vi "rtc.vi"(8 "per":dbl, 9 "Altitude (Z)":dbl(slide)=2.0 scale=0.0..10.0, 10 "Longitude (Y)":dbl(slide) scale=0.0..10.0, 11 "Latitude (X)":dbl(slide)) -> (0 "yaw":dbl, 1 "Zo":dbl, 2 "Yo":dbl, 3 "Xo":dbl, 4 "pitch":dbl, 6 "h":dbl)   [LabVIEW 2015]
uses:
  <vilib>/imath/engines/lvmath2/RunTimeEngine/Managers/WorkSpace/UID Generator.vi
  <vilib>/imath/engines/lvmath2/RunTimeEngine/BuiltInFunctions/pause/NIMS_pause(S).vi
  <vilib>/imath/engines/lvmath2/RunTimeEngine/RunTimeType/NIMS_RunTimeType_From StrictType (excl LVString).vi
  <instcachedir>/0/NIMS_RunTimeType_From StrictType (excl LVString)_EB1C38A9BC5048DA9ABDA8F781E54D21.lvgen/NIMS_RunTimeType_From StrictType (excl LVString)_EB1C38A9BC5048DA9ABDA8F781E54D21_000.vi
  <vilib>/imath/engines/lvmath2/RunTimeEngine/LocalVariableDefStatement/MC_LocalVariableDefStatement_Display.vi
  <vilib>/imath/engines/lvmath2/RunTimeEngine/Managers/SymbolTable/Clear UID.vi
  <vilib>/imath/engines/lvmath2/RunTimeEngine/NodeEndStatement/NIMS_NodeEndStatement_Output.vi
  <instcachedir>/0/NIMS_NodeEndStatement_Output_53EC0D466D134D7ABD903AC30B43404B.lvgen/NIMS_NodeEndStatement_Output_53EC0D466D134D7ABD903AC30B43404B_001.vi
  <vilib>/imath/engines/lvmath2/RunTimeEngine/ErrorHandling/NIMS_Finalize Error.vi
  <vilib>/imath/engines/lvmath2/RunTimeEngine/Managers/SymbolTable/NIMS_WorkSpace.lvlib
panel:
  in  "time":dbl=0.001
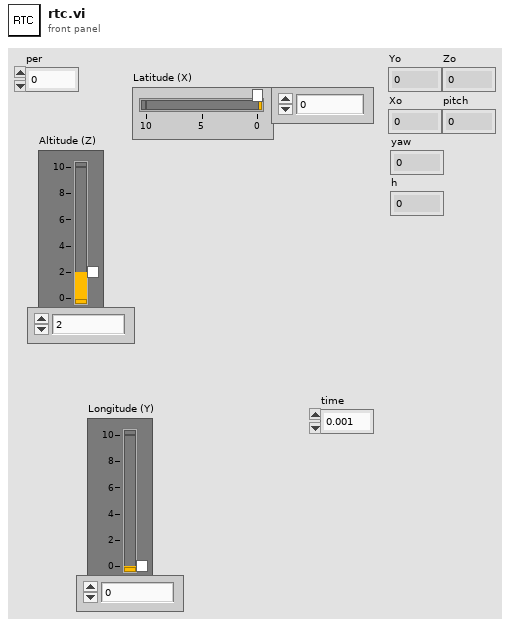
[diagram p1: front panel]
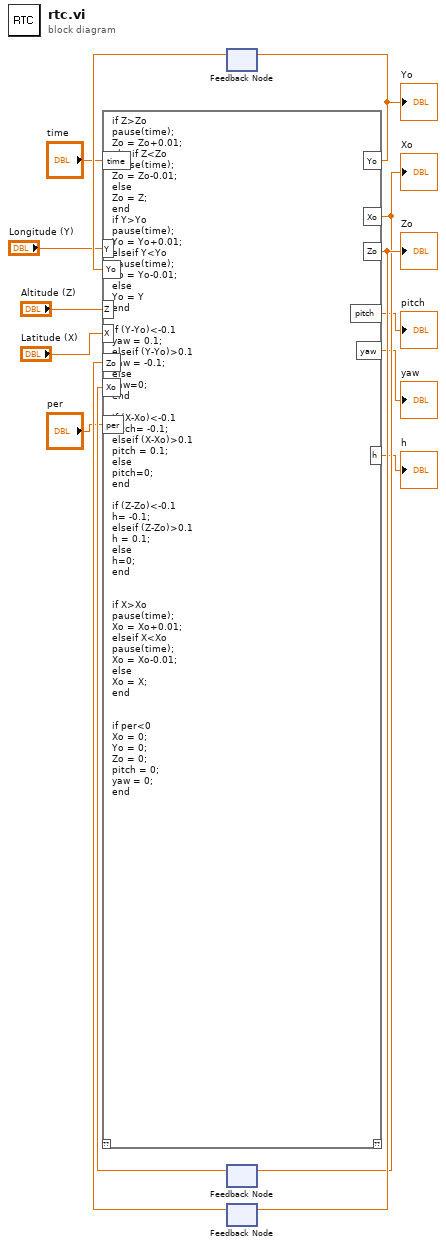
[diagram p0: block diagram]
diagram:
  n1 = feedback #1() -> (w13:dbl)  [unwired: 1 in]
  n2 = feedback #2() -> (w9:dbl)  [unwired: 1 in]
  n3 = feedback #3() -> (w8:dbl)  [unwired: 1 in]
  n4 = mathscript code="if Z>Zo\npause(time);\nZo = Zo+0.01;\nelseif Z<Zo\npause(time);\nZo = Zo-0.01;\nelse\nZo = Z;\nend\nif Y>Yo\npause(time);\nYo = Yo+0.01;\nelseif Y<Yo\npause(time);\nYo = Yo-0.01;\nelse\nYo = Y\nend\n\nif (Y-Yo)<-0.1\nyaw = 0.1;\nelseif (Y-Yo)>0.1\nyaw = -0.1;\nelse\nyaw=0;\nend\n\nif (X-Xo)<-0.1\npitch= -0.1;\nelseif (X-Xo)>0.1\npitch = 0.1;\nelse\npitch=0;\nend\n\nif (Z-Zo)<-0.1\nh= -0.1;\nelseif (Z-Zo)>0.1\nh = 0.1;\nelse\nh=0;\nend\n\n\nif X>Xo\npause(time);\nXo = Xo+0.01;\nelseif X<Xo\npause(time);\nXo = Xo-0.01;\nelse\nXo = X;\nend\n\n\nif per<0\nXo = 0;\nYo = 0;\nZo = 0;\npitch = 0;\nyaw = 0;\nend"("Y"="Longitude (Y)", "Yo"=w13, "time"="time", "Z"="Altitude (Z)", "X"="Latitude (X)", "Zo"=w8, "Xo"=w9, "per"="per") -> ("Yo"=w14:dbl, "Xo"=w10:dbl, "Zo"=w11:dbl, "pitch"=→"pitch":dbl, "yaw"=→"yaw":dbl, "h"=→"h":dbl)  [unwired: 1 in, 1 out]
  "Yo" <- w14
  "Xo" <- w10
  "Zo" <- w11
  n5 = feedback-in #1 ("2")(w14) -> ()
  n6 = feedback-in #2(w10) -> ()
  n7 = feedback-in #3(w11) -> ()
